vi "Insert Left SubPanel.vi"(8 "error in (no error)":errorcluster, 9 "ActorQName":string, 10 "ActorVI Ref":refnum<vi>, 11 "CallActorCenter in":refnum<class "CallActorCenter.lvclass">) -> (0 "error out":errorcluster, 3 "CallActorCenter out":refnum<class "CallActorCenter.lvclass">)   [LabVIEW 2021, in "CallActorCenter.lvclass"]
uses:
  CallActorCenter.lvclass
  CallActorCenter.lvclass/CallActorCenter.ctl
  <userlib>/John_Lib/Interfaces/InsertLeftSubPanel/InsertLeftSubPanel Messages/Insert Left SubPanel Msg/Insert Left SubPanel Msg.lvclass
  <userlib>/John_Lib/AbstractActorTemplate/AbstractActorTemplate/UIActorTop.lvclass
  C:/Program Files (x86)/National Instruments/LabVIEW 2021/user.lib/John_Lib/AbstractActorTemplate/AbstractActorTemplate/UIActorTop.lvclass
  C:/Program Files (x86)/National Instruments/LabVIEW 2021/vi.lib/ActorFramework/Actor/Actor.lvclass
  C:/Program Files (x86)/National Instruments/LabVIEW 2021/project/Create Actor from Template/_CallActorCenter/CallActorCenter.lvclass
  C:/Program Files (x86)/National Instruments/LabVIEW 2021/user.lib/John_Lib/Interfaces/CheckPassWord/CheckPassWord.lvclass
  C:/Program Files (x86)/National Instruments/LabVIEW 2021/user.lib/John_Lib/Interfaces/FrontPanel Save Image/FrontPanel Save Image.lvclass
  C:/Program Files (x86)/National Instruments/LabVIEW 2021/user.lib/John_Lib/Interfaces/InsertButtonSubPanel/InsertButtonSubPanel.lvclass
  C:/Program Files (x86)/National Instruments/LabVIEW 2021/user.lib/John_Lib/Interfaces/InsertLeftSubPanel/InsertLeftSubPanel.lvclass
  C:/Program Files (x86)/National Instruments/LabVIEW 2021/user.lib/John_Lib/Interfaces/InsertMainSubPanel/InsertMainSubPanel.lvclass
  C:/Program Files (x86)/National Instruments/LabVIEW 2021/user.lib/John_Lib/Interfaces/InsertRightSubPanel/InsertRightSubPanel.lvclass
  C:/Program Files (x86)/National Instruments/LabVIEW 2021/user.lib/John_Lib/Interfaces/InsertSubPanel/InsertSubPanel.lvclass
  C:/Program Files (x86)/National Instruments/LabVIEW 2021/user.lib/John_Lib/Interfaces/Windows Title/Windows Title.lvclass
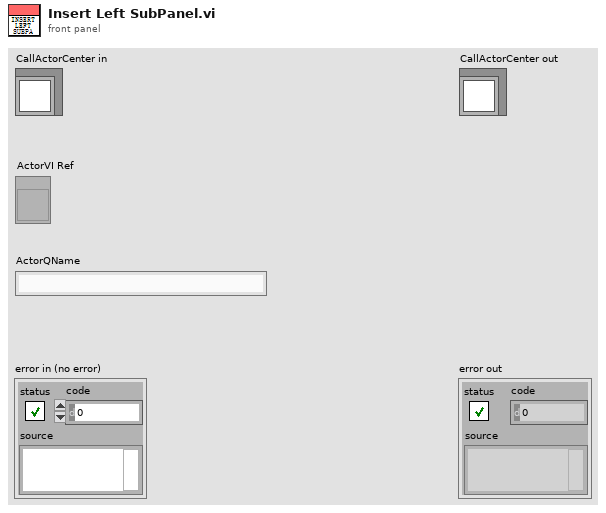
[diagram p1: front panel]
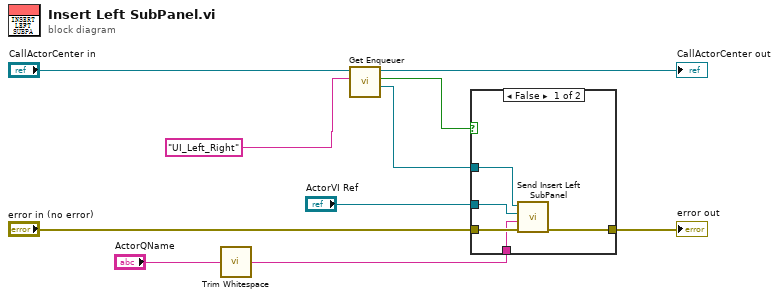
[diagram p0: block diagram]
diagram:
  n1 = call <vilib>:"Trim Whitespace.vi"("string"="ActorQName") -> ("trimmed string"=w6:string)  [unwired: 1 in]
  n2 = call <userlib>:"Get Enqueuer.vi"("ActorQName"="UI_Left_Right" ("key"), "UIActorTop in"="CallActorCenter in") -> ("Nested Actor's Enqueuer"=w1:refnum<class "Message Enqueuer.lvclass">, "key not found?"=w2:bool, "UIActorTop out"=→"CallActorCenter out":refnum<class "CallActorCenter.lvclass">)  [unwired: 3 in, 4 out]
  n3 = case shown="False" w2 {
    tunnel: w1 -> [w15 _]
    tunnel: "ActorVI Ref" -> [w14 _]
    tunnel: "error in (no error)" -> [w13 w16]
    tunnel: [w12 w16] -> w9
    tunnel: w6 -> [w11 _]
    frame False {
      n4 = call <userlib>:"Send Insert Left SubPanel.vi"("error in (no error)"=w13, "ActorQName"=w11, "ActorVI Ref"=w14, "Message Enqueuer"=w15) -> ("error out"=w12:errorcluster)  [unwired: 6 in, 1 out]
    }
    frame True {
    }
  }
  "error out" <- w9
